vi "st_eval CDF (f).vi"(4 "parameters":variant, 5 "x":dbl) -> (2 "f(x)":dbl)   [LabVIEW 2017, in "NI_Gmath.lvlib"]
uses:
  NI_Gmath.lvlib
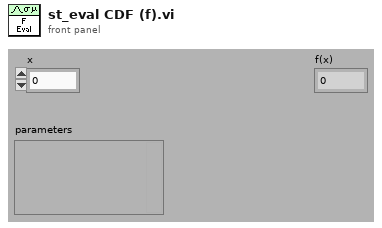
[diagram p1: front panel]
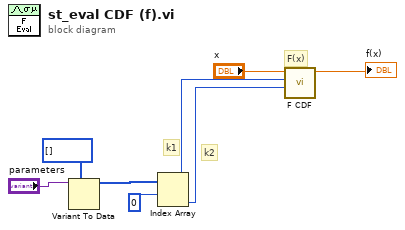
[diagram p0: block diagram]
diagram:
  # "k2"
  # "k1"
  # "F(x)"
  n1 = Variant To Data(type=i32[] [], Variant="parameters") -> (data=w6:i32[])  [unwired: 1 in, 1 out]
  n2 = Index Array(array=w6, index #1=0 ("index")) -> (element #1=w1:i32, element #2=w3:i32)  [unwired: 1 in]
  n3 = call "F CDF.vi"("k2"=w3, "k1"=w1, "x"="x") -> ("cdf(x)"=→"f(x)":dbl)  [unwired: 7 in, 1 out]
